vi "SpeedAccelDistanceM1M2.vi"(4 "Distance1":u32 max=127 step=1, 5 "Speed2":i32 max=127 step=1, 6 "Immediate":u8 max=127 step=1, 7 "Accel":u32 max=127 step=1, 8 "error in (no error)":errorcluster, 9 "Address":u8=46, 10 "Speed1":i32 max=127 step=1, 11 "VISA Refnum in":refnum<visa-resource-name>) -> (0 "error out":errorcluster, 2 "Valid":bool, 3 "VISA Refnum out":refnum<visa-resource-name>)   [LabVIEW 2015, in "Ion Motion Roboclaw.lvlib"]
uses:
  <instrlib>/Ion Motion Roboclaw/Ion Motion Roboclaw.lvlib
panel:
  in  "Distance2":u32 max=127 step=1
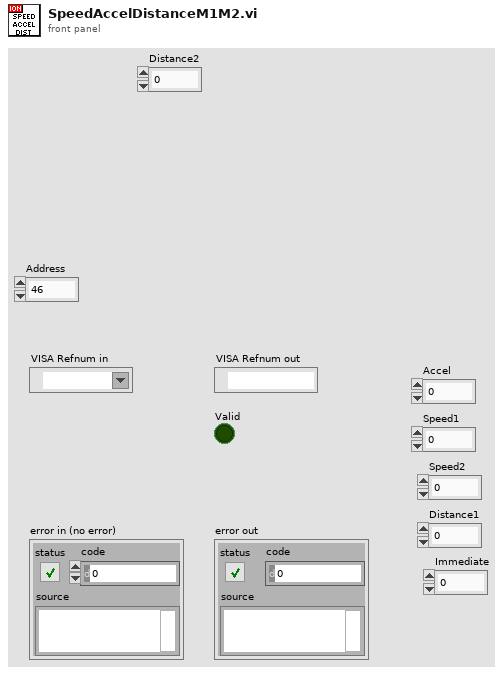
[diagram p1: front panel]
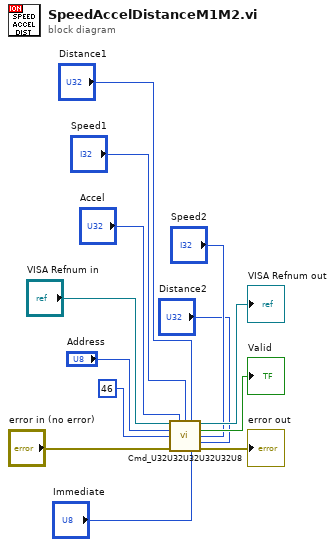
[diagram p0: block diagram]
diagram:
  n1 = call <instrlib>:"Cmd_U32U32U32U32U32U8.vi"("VISA Refnum in"="VISA Refnum in", "Arg1"="Accel", "Arg2"="Speed1", "Arg3"="Distance1", "Address"="Address", "Cmd"=u8 46, "Arg4"="Speed2", "Arg5"="Distance2", "error in (no error)"="error in (no error)", "Arg6"="Immediate") -> ("VISA Refnum out"=→"VISA Refnum out":refnum<visa-resource-name>, "Valid"=→"Valid":bool, "error out"=→"error out":errorcluster)  [unwired: 3 in]
